vi "Create Message Setter.vi"(7 "RPC Message Name":string, 8 "error in (no error)":errorcluster, 11 "RPC Messages Folder (ProjectItem) in":refnum<vi>) -> (0 "error out":errorcluster, 2 "Message Setter out":refnum<vi>, 3 "RPC Messages Folder (ProjectItem) out":refnum<vi>)   [LabVIEW 2019, in "gRPC Template Creation Utility.lvlib"]
uses:
  gRPC Template Creation Utility.lvlib
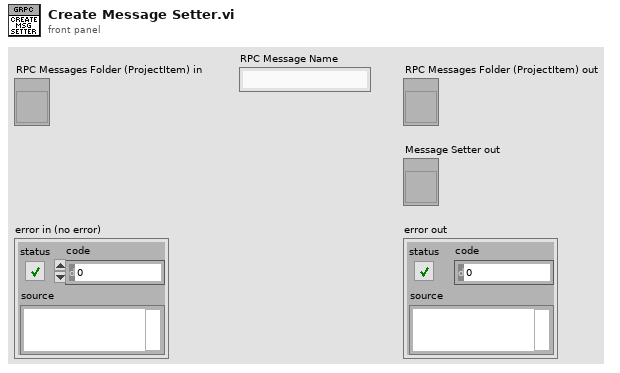
[diagram p1: front panel]
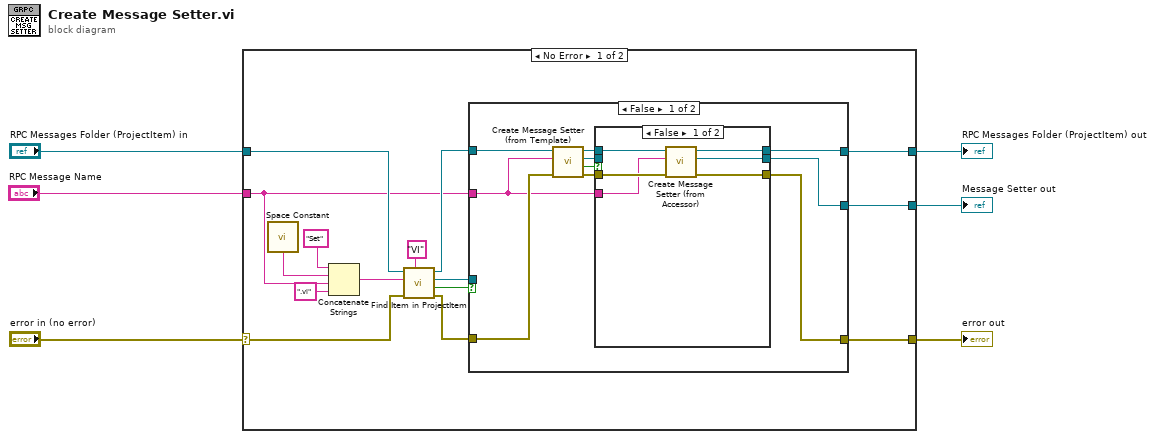
[diagram p0: block diagram]
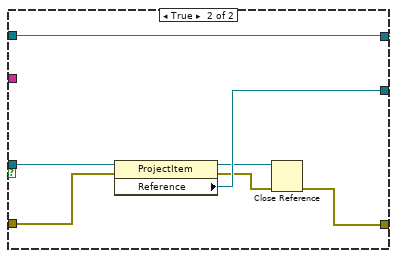
[diagram p3: hidden frame]
diagram:
  n1 = case shown="No Error" "error in (no error)" {
    selector: "error in (no error)" -> [w15 w49]
    tunnel: [w9 w48] -> w6
    tunnel: [w7 w49] -> w5
    tunnel: "RPC Messages Folder (ProjectItem) in" -> [w20 w48]
    tunnel: "RPC Message Name" -> [w11 _]
    tunnel: [w8 _] -> w1
    frame No Error {
      n2 = call <vilib>:"Space Constant.vi"() -> ("String"=w18:string)
      n3 = Concatenate Strings("Set" ("string"), w18, w11, ".vi" ("string")) -> (w16:string)
      n4 = call "Find Item in ProjectItem.vi"("Item Type"="VI", "error in (no error)"=w15, "Name"=w16, "ProjectItem in"=w20) -> ("error out"=w10:errorcluster, "Found ?"=w13:bool, "Item Refnum out"=w12:refnum<vi>, "ProjectItem out"=w14:refnum<vi>)  [unwired: 4 in]
      n5 = case shown="False" w13 {
        tunnel: [w30 w46] -> w8
        tunnel: [w31 w45] -> w9
        tunnel: w10 -> [w27 w41]
        tunnel: [w29 w42] -> w7
        tunnel: w14 -> [w28 w45]
        tunnel: w12 -> [_ w47]
        tunnel: w11 -> [w22 _]
        frame False {
          n6 = call "Create Message Setter (from Template).vi"("error in (no error)"=w27, "RPC Message Name"=w22, "RPC Messages Folder (ProjectItem) in"=w28) -> ("error out"=w23:errorcluster, "Created?"=w24:bool, "VI out"=w25:refnum<vi>, "RPC Messages Folder (ProjectItem) out"=w26:refnum<vi>)  [unwired: 5 in]
          n7 = case shown="False" w24 {
            tunnel: w23 -> [w36 w39]
            tunnel: w26 -> [w37 w40]
            tunnel: w25 -> [_ w38]
            tunnel: [w34 w40] -> w31
            tunnel: [w32 w39] -> w29
            tunnel: [w33 w38] -> w30
            tunnel: w22 -> [w35 _]
            frame False {
              n8 = call "Create Message Setter (from Accessor).vi"("error in (no error)"=w36, "RPC Message Name"=w35, "RPC Messages Folder (ProjectItem) in"=w37) -> ("error out"=w32:errorcluster, "Getter VI out"=w33:refnum<vi>, "RPC Messages Folder (ProjectItem) out"=w34:refnum<vi>)  [unwired: 5 in, 1 out]
            }
            frame True {
            }
          }
        }
        frame True {
          n9 = property class="ProjectItem"(reference=w47, error in=w41) -> (reference out=w43:refnum<vi>, error out=w44:errorcluster, "Reference"=w46:refnum<vi>)
          n10 = Close Reference(reference=w43, error in (no error)=w44) -> (error out=w42:errorcluster)
        }
      }
    }
    frame Error {
    }
  }
  "error out" <- w5
  "Message Setter out" <- w1
  "RPC Messages Folder (ProjectItem) out" <- w6
